vi "ACQ Setup.vi"(6 "End Index":i16=-1, 8 "error in (no error)":errorcluster, 9 "Start Index":i16, 10 "Sensor 2":bool, 11 "Sensor 1":bool) -> (0 "error out":errorcluster)   [LabVIEW 2015, in "Tool Interface.lvlib"]
uses:
  Tool Interface.lvlib
  Tool Typedefs/_ACQ Setup Params Cluster--typedef.ctl
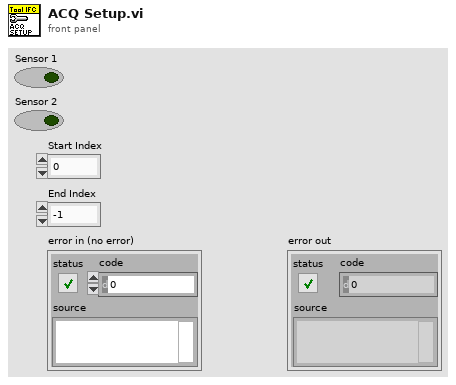
[diagram p1: front panel]
types:
  T1 = typedef "_ACQ Setup Params Cluster--typedef.ctl" = cluster{"Sensor 1":bool, "Sensor 2":bool, "Start Index":u16, "End Index":u16}
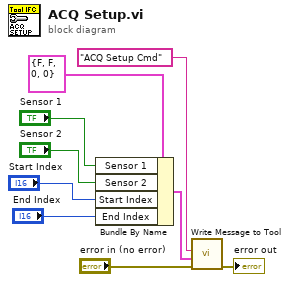
[diagram p0: block diagram]
diagram:
  n1 = Bundle By Name(cluster=T1 {"Sensor 1"=FALSE, "Sensor 2"=FALSE, "Start Index"=0, "End Index"=0} ("_Laser Params Cluster--typedef"), "Sensor 1"="Sensor 1", "Sensor 2"="Sensor 2", "Start Index"="Start Index", "End Index"="End Index") -> (w8:T1)
  n2 = call "Write Message to Tool.vi"("error in (no error)"="error in (no error)", "Message Data"=w8, "Message"="ACQ Setup Cmd") -> ("error out"=→"error out":errorcluster)  [unwired: 8 in]
